vi "Copy InstrumentStudio Plug-In Data File.vi"(0 "configuration":T1, 5 "Plugin Path":path, 11 "error in":errorcluster) -> (4 "G Plugin Data File Path":path, 15 "error out":errorcluster)   [LabVIEW 2021, in "InstrumentStudio Plug-In Editor.lvlib"]
uses:
  InstrumentStudio Plug-In Editor.lvlib
  controls/Data Holder.ctl
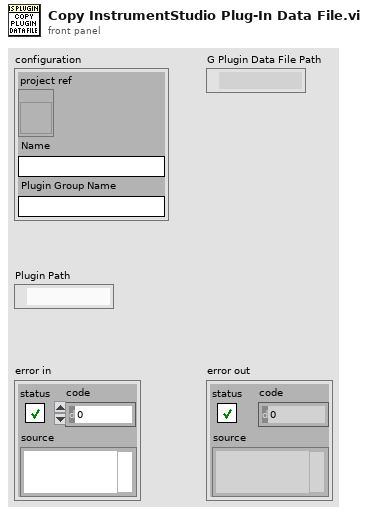
[diagram p1: front panel]
types:
  T1 = typedef "InstrumentStudio Plug-In Editor.lvlib/Data Holder.ctl" = cluster{"project ref":refnum<vi>, "Name":string, "Plugin Group Name":string}
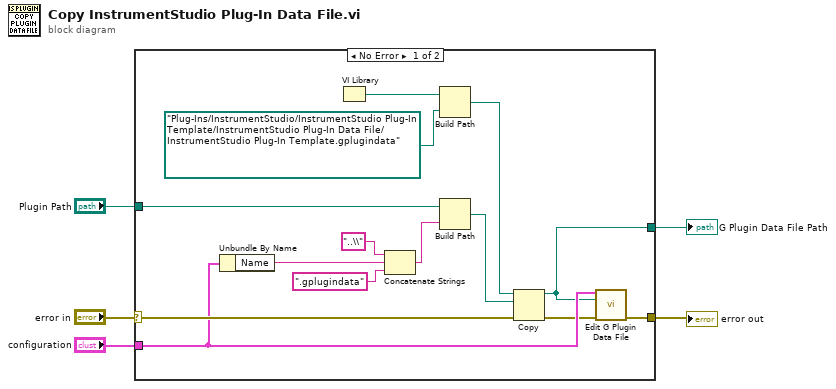
[diagram p0: block diagram]
diagram:
  n1 = case shown="No Error" "error in" {
    selector: "error in" -> [w19 w20]
    tunnel: [w14 w20] -> w5
    tunnel: "Plugin Path" -> [w16 _]
    tunnel: "configuration" -> [w15 _]
    tunnel: [w6 _] -> w1
    frame No Error {
      n2 = Unbundle By Name(w15) -> ("Name"=w9:string)
      n3 = VI Library() -> (path=w10:path)
      n4 = Concatenate Strings("..\\" ("string"), w9, ".gplugindata" ("string")) -> (w17:string)
      n5 = Build Path(base path=w10, name or relative path=path "Plug-Ins/InstrumentStudio/InstrumentStudio Plug-In Template/InstrumentStudio Plug-In Data File/InstrumentStudio Plug-In Template.gplugindata") -> (appended path=w12:path)
      n6 = Build Path(base path=w16, name or relative path=w17) -> (appended path=w18:path)
      n7 = Copy(8:w19, 10:w18, 11:w12) -> (0:w13:errorcluster, 3:w6:path)  [unwired: 2 in, 1 out]
      n8 = call "Edit G Plugin Data File.vi"("configuration"=w15, "Path"=w6, "error in"=w13) -> ("error out"=w14:errorcluster)  [unwired: 12 in]
    }
    frame Error {
    }
  }
  "error out" <- w5
  "G Plugin Data File Path" <- w1
